vi "Pose Distance.vi"(10 "Pose2d 2":T1, 11 "Pose2d":T1) -> (3 "Distance":dbl)   [LabVIEW 2019]
uses:
  Typedef/Pose2d.ctl
  Typedef/Translation2d.ctl
  Typedef/Rotation2d.ctl
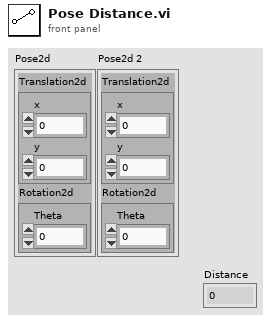
[diagram p1: front panel]
types:
  T1 = typedef "Pose2d.ctl" = cluster{"Translation2d":T2, "Rotation2d":T3}
  T2 = typedef "Translation2d.ctl" = cluster{"x":dbl, "y":dbl}
  T3 = typedef "Rotation2d.ctl" = cluster{"Theta":dbl}
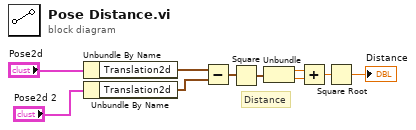
[diagram p0: block diagram]
diagram:
  # "Distance"
  n1 = Unbundle By Name("Pose2d") -> ("Translation2d"=w4:T2)
  n2 = Unbundle By Name("Pose2d 2") -> ("Translation2d"=w2:T2)
  n3 = Subtract(x=w4, y=w2) -> (x-y=w9:T2)
  n4 = Square(x=w9) -> (x^2=w10:T2)
  n5 = Unbundle(w10) -> ("x"=w5:dbl, "y"=w6:dbl)
  n6 = Add(x=w5, y=w6) -> (x+y=w7:dbl)
  n7 = Square Root(x=w7) -> (sqrt(x)=→"Distance":dbl)
